vi "Handle TCP Message.vi"(7 "TCPMessageAPI":refnum<class "TCPMessageAPI.lvclass">, 8 "error in (no error)":errorcluster, 10 "TcpPayload":T1, 11 "RequestReply Message Handler in":refnum<class "RequestReply Message Handler.lvclass">) -> (0 "error out":errorcluster, 3 "RequestReply Message Handler out":refnum<class "RequestReply Message Handler.lvclass">)   [LabVIEW 2020, in "VectoScratch.lvlib" / "RequestReply Message Handler.lvclass"]
uses:
  RequestReply Message Handler.lvclass
  Vecto/TCPMessageService/TCPMessageAPI.lvclass
  Vecto/proto/TcpPayload/Data.ctl
  Vecto/proto/TcpPayload/TcpPayload.lvlib
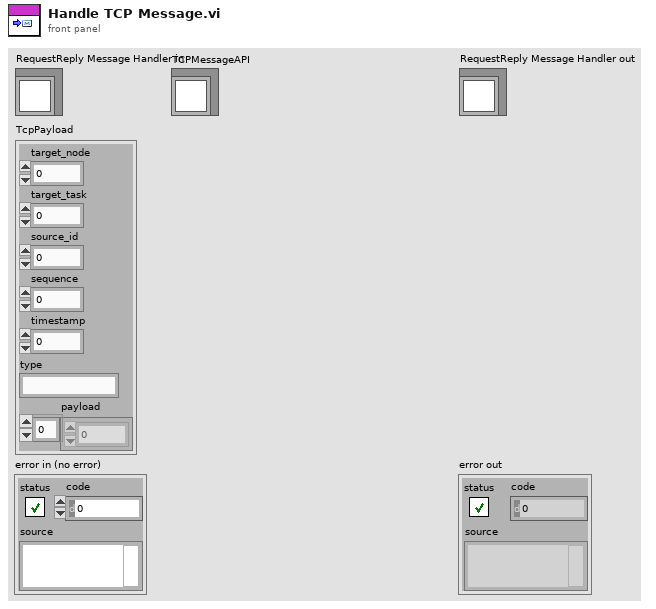
[diagram p1: front panel]
types:
  T1 = typedef "TcpPayload.lvlib/Data.ctl" = cluster{"target_node":u32, "target_task":u32, "source_id":u32, "sequence":u32, "timestamp":u64, "type":string, "payload":u8[]}
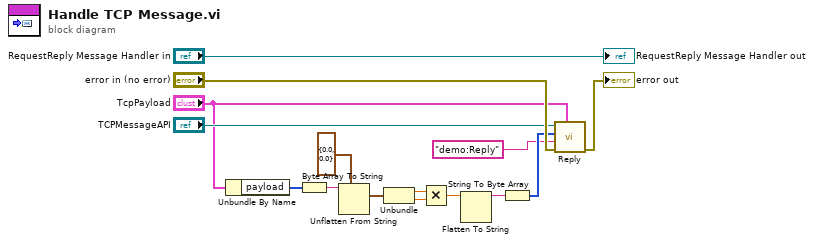
[diagram p0: block diagram]
diagram:
  n1 = Unbundle By Name("TcpPayload") -> ("payload"=w13:u8[])
  n2 = Byte Array To String(unsigned byte array=w13) -> (string=w12:string)
  n3 = Unflatten From String(type=cluster{dbl, dbl} {0.0, 0.0}, binary string=w12) -> (value=w4:cluster{dbl, dbl})  [unwired: 3 in, 2 out]
  n4 = Unbundle(w4) -> (w10:dbl, w9:dbl)
  n5 = Multiply(x=w10, y=w9) -> (x*y=w2:dbl)
  n6 = Flatten To String(anything=w2) -> (data string=w8:string)  [unwired: 3 in, 2 out]
  n7 = String To Byte Array(string=w8) -> (unsigned byte array=w5:u8[])
  n8 = call "Reply.vi"("Original Payload"="TcpPayload", "error in (no error)"="error in (no error)", "Type"="demo:Reply", "Payload"=w5, "TCPMessageAPI in"="TCPMessageAPI") -> ("error out"=→"error out":errorcluster)  [unwired: 5 in, 1 out]
  "RequestReply Message Handler out" <- "RequestReply Message Handler in"
